vi "Solve2.vi"(8 "Error In":errorcluster, 11 "object in":refnum<class "2021_13.lvclass">) -> (0 "Error Out":errorcluster, 2 "Result":u64, 3 "object out":refnum<class "2021_13.lvclass">)   [LabVIEW 2020, in "2021_13.lvclass"]
uses:
  2021_13.lvclass
  2021_13.lvclass/2021_13.ctl
panel:
  out "Array":bool[][](array[boolean])
  # "JKZBLQKA\nJRZBLQKH"
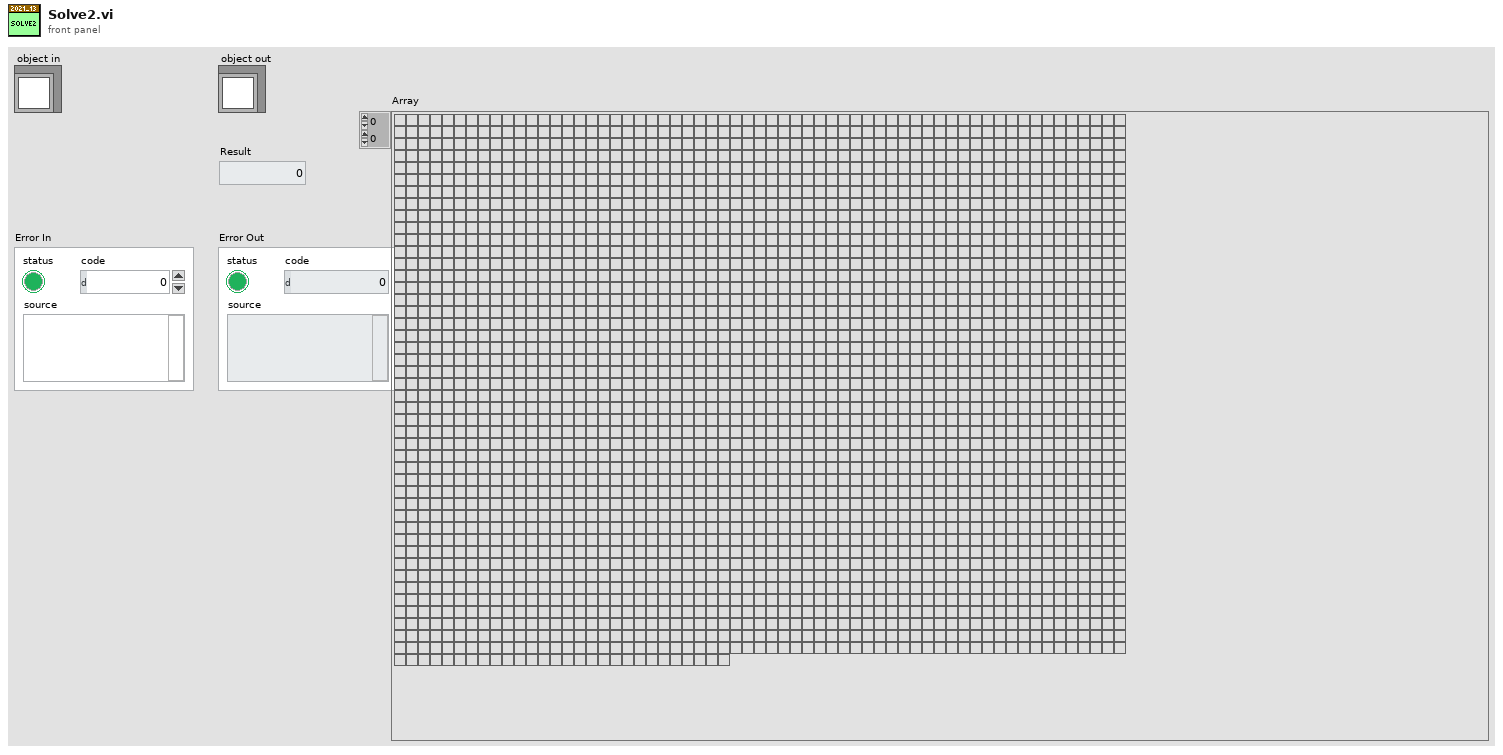
[diagram p1: front panel]
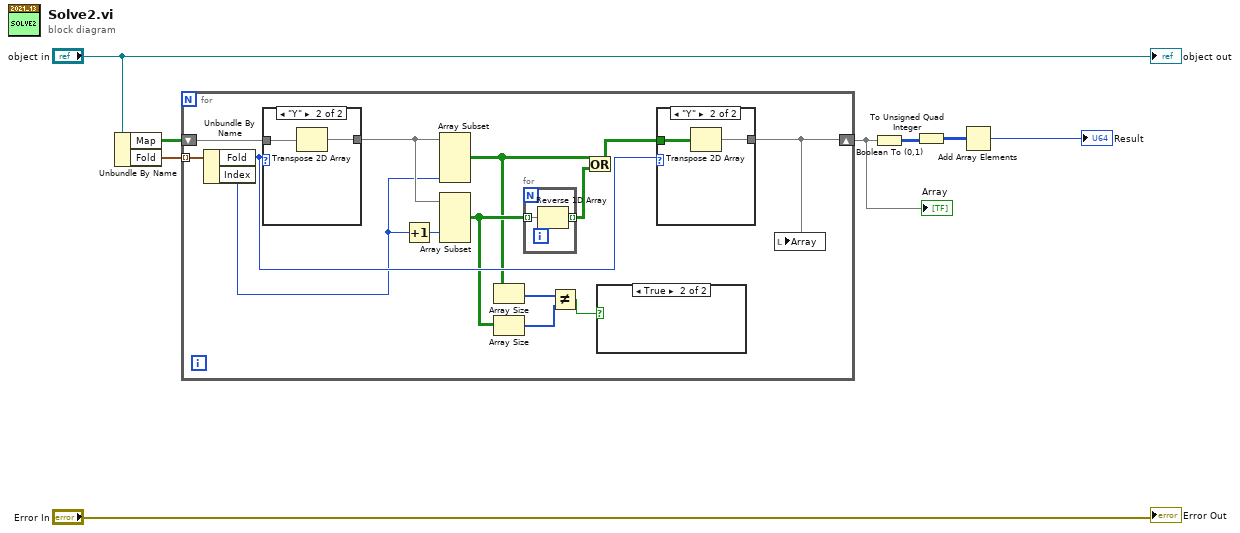
[diagram p0: block diagram]
diagram:
  n1 = Unbundle By Name("object in") -> ("Map"=w5:bool[][], "Fold"=w6:cluster{"Fold":enum16{"X", "Y"}, "Index":i32}[])
  n2 = for {
    tunnel: w6 -> [w22] mode=indexing
    shift-right: [w14] -> w1
    shift-left: w5 -> [w21]
    n3 = Unbundle By Name(w22) -> ("Fold"=w20:enum16{"X", "Y"}, "Index"=w18:i32)
    n4 = case shown="\"Y\"" w20 {
      tunnel: w21 -> [w28 w30]
      tunnel: [w28 w29] -> w19
      frame "X", Default {
      }
      frame "Y" {
        n5 = Transpose 2D Array(2D array=w30) -> (transposed array=w29:bool[][])
      }
    }
    n6 = Increment(x=w18) -> (x+1=w17:i32)
    n7 = Array Subset(array=w19, length (col)=w18) -> (w12:bool[][])  [unwired: 3 in]
    n8 = Array Subset(array=w19, index (col)=w17) -> (w13:bool[][])  [unwired: 3 in]
    n9 = Array Size(array=w12) -> (size(s)=w11:i32[])
    n10 = Array Size(array=w13) -> (size(s)=w10:i32[])
    n11 = for {
      tunnel: w13 -> [w24] mode=indexing
      tunnel: [w23] -> w16 mode=indexing
      n12 = Reverse 1D Array(array=w24) -> (reversed array=w23:bool[])
    }
    n13 = Not Equal?(x=w11, y=w10) -> (x != y?=w9:bool)
    n14 = Or(x=w12, y=w16) -> (x .or. y?=w15:bool[][])
    n15 = case shown="True" w9 {
      frame False {
      }
      frame True {
      }
    }
    n16 = case shown="\"Y\"" w20 {
      tunnel: w15 -> [w25 w27]
      tunnel: [w25 w26] -> w14
      frame "X", Default {
      }
      frame "Y" {
        n17 = Transpose 2D Array(2D array=w27) -> (transposed array=w26:bool[][])
      }
    }
    n18 = local write "Array"(w14) -> ()
  }
  "Array" <- w1
  n19 = Boolean To (0,1)(Boolean=w1) -> (0, 1=w4:i16[][])
  n20 = To Unsigned Quad Integer(1:w4) -> (0:w3:u64[][])
  n21 = Add Array Elements(numeric array=w3) -> (sum=→"Result":u64)
  "Error Out" <- "Error In"
  "object out" <- "object in"
